vi "DeviceOff.vi"(8 "error in (no error)":errorcluster, 11 "ChromaAcLoad in":refnum<class "ChromaAcLoad.lvclass">) -> (0 "error out":errorcluster, 3 "ChromaAcLoad out":refnum<class "ChromaAcLoad.lvclass">)   [LabVIEW 2018, in "AcPwrPlugins.lvlib" / "ChromaAcLoad.lvclass"]
uses:
  ChromaAcLoad.lvclass
  C:/Users/ico/Documents/Projects/NistPluggableModules/AcPwr/AcPwrPlugins/AcPwrBaseClass/AcPwrBase.lvclass
  AcPwrBaseClass/AcPwrBase.lvclass/AcPwrBase.ctl
  AcPwrBaseClass/Accessors/Read BaseConfig.vi
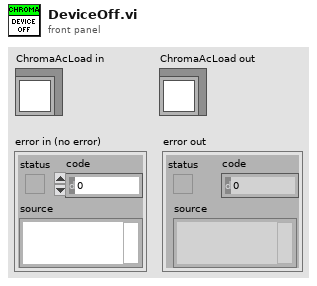
[diagram p1: front panel]
types:
  T1 = typedef "AcPwrPlugins.lvlib/AcPwrBase.lvclass/BaseConfig.ctl" = cluster{"Frequency":dbl, "FrequencyRange":dbl[], "Phases":T2[]}
  T2 = typedef "AcPwrPlugins.lvlib/AcPwrBase.lvclass/Phase.ctl" = cluster{"Enabled":bool, "VoltageLevel":dbl, "Waveform":string, "Name":string, "VoltageRange":dbl[], "CurrentLimit":dbl, "Handle":string, "Connected":bool}
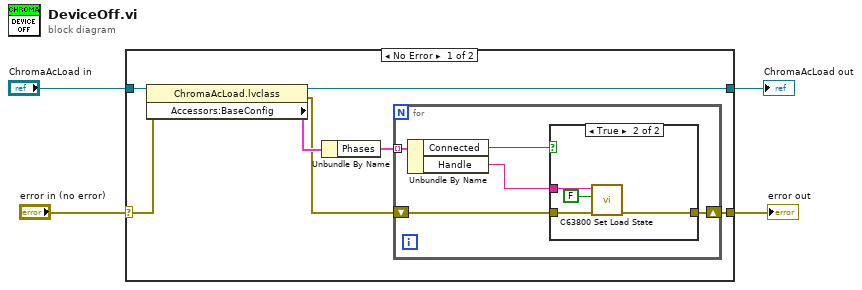
[diagram p0: block diagram]
diagram:
  n1 = case shown="No Error" "error in (no error)" {
    selector: "error in (no error)" -> [w10 w23]
    tunnel: [w7 w23] -> w2
    tunnel: [w11 w22] -> w1
    tunnel: "ChromaAcLoad in" -> [w5 w22]
    frame No Error {
      n2 = property class="ChromaAcLoad.lvclass"(reference=w5, error in=w10) -> (reference out=w11:refnum<class "ChromaAcLoad.lvclass">, error out=w6:errorcluster, "Accessors:BaseConfig"=w9:T1)
      n3 = Unbundle By Name(w9) -> ("Phases"=w8:T2[])
      n4 = for {
        tunnel: w8 -> [w16] mode=indexing
        shift-right: [w15] -> w7
        shift-left: w6 -> [w12]
        n5 = Unbundle By Name(w16) -> ("Connected"=w13:bool, "Handle"=w14:string)
        n6 = case shown="True" w13 {
          tunnel: [w17 w21] -> w15
          tunnel: w12 -> [w17 w18]
          tunnel: w14 -> [_ w19]
          frame False {
          }
          frame True, Default {
            n7 = call <instrlib>:"C63800 Set Load State.vi"("error in (no error)"=w18, "Load State"=FALSE ("Output Enabled (False)"), "Instrument Handle"=w19) -> ("error out"=w21:errorcluster)  [unwired: 7 in, 1 out]
          }
        }
      }
    }
    frame Error {
    }
  }
  "error out" <- w2
  "ChromaAcLoad out" <- w1
